vi "CPF_fast.vi"(1 "y":dbl=1.0, 2 "x":dbl=1.0) -> (0 "CPF Value":cdb=0.3047442052569335+0.2082189382028505i format="%#_12g")   [LabVIEW 2015]
panel:
  # "CPF algorithm"
  # "Fast CPF algorithm:\n  Computes the complex probability function using Humlicek's algorithm in\n  its first subregion (Source: 10.1016/0022-4073(82)90078-4) and using a\n  rational series with 24 terms in other subregions. (Source: \n  jstor.org/stable/2158232)\n\nStandard Input Parameters:\n-------------------- \nx  : Real part of input complex parameter\ny  : Imaginary part of input complex parameter\n\nThe function has one output:\n--------------------\n(1): Complex probability function"
  # "Output Section"
  # "Input Section"
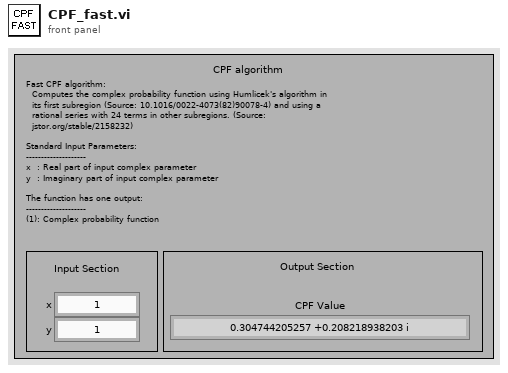
[diagram p1: front panel]
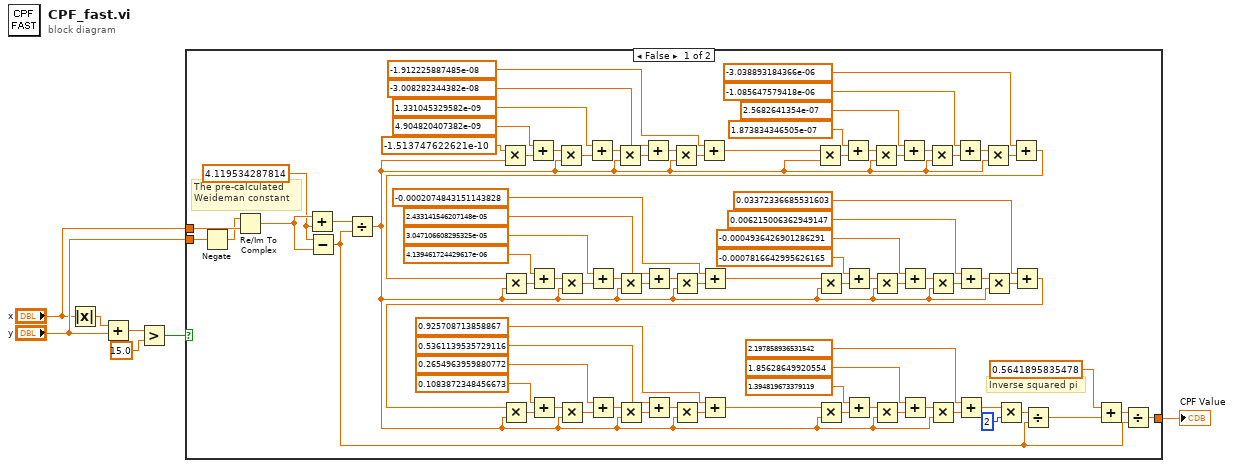
[diagram p0: block diagram]
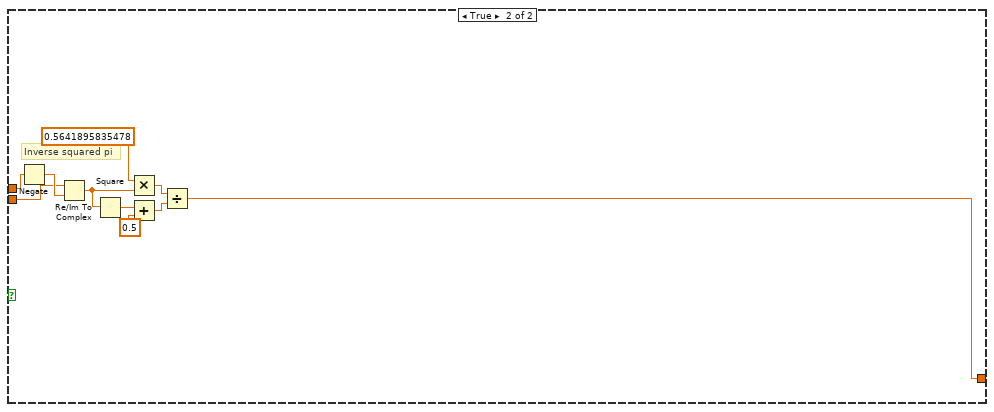
[diagram p2: hidden frame]
diagram:
  n1 = Absolute Value(x="x") -> (abs(x)=w4:dbl)
  n2 = Add(x=w4, y="y") -> (x+y=w3:dbl)
  n3 = Greater?(x=w3, y=15.0) -> (0:w5:bool)
  n4 = case shown="False" w5 {
    tunnel: "x" -> [w90 w101]
    tunnel: "y" -> [w91 w99]
    tunnel: [w77 w93] -> w1
    frame False {
      w87 = 4.119534287814 ("L")
      # "Inverse squared pi"
      # "The pre-calculated \nWeideman constant"
      n5 = Negate(x=w91) -> (-x=w89:dbl)
      n6 = Re/Im To Complex(1:w90, 2:w89) -> (0:w88:cdb)
      n7 = Add(x=w88, y=w87) -> (x+y=w86:cdb)
      n8 = Subtract(x=w87, y=w88) -> (x-y=w78:cdb)
      n9 = Divide(x=w86, y=w78) -> (x/y=w85:cdb)
      n10 = Multiply(x=-1.513747622621e-10, y=w85) -> (x*y=w76:cdb)
      n11 = Add(x=4.904820407382e-09, y=w76) -> (x+y=w75:cdb)
      n12 = Multiply(x=w75, y=w85) -> (x*y=w73:cdb)
      n13 = Add(x=1.331045329582e-09, y=w73) -> (x+y=w74:cdb)
      n14 = Multiply(x=w74, y=w85) -> (x*y=w70:cdb)
      n15 = Add(x=-3.008282344382e-08, y=w70) -> (x+y=w72:cdb)
      n16 = Multiply(x=w72, y=w85) -> (x*y=w71:cdb)
      n17 = Add(x=-1.912225887485e-08, y=w71) -> (x+y=w62:cdb)
      n18 = Multiply(x=w62, y=w85) -> (x*y=w69:cdb)
      n19 = Add(x=1.873834346505e-07, y=w69) -> (x+y=w68:cdb)
      n20 = Multiply(x=w68, y=w85) -> (x*y=w66:cdb)
      n21 = Add(x=2.5682641354e-07, y=w66) -> (x+y=w67:cdb)
      n22 = Multiply(x=w67, y=w85) -> (x*y=w63:cdb)
      n23 = Add(x=-1.085647579418e-06, y=w63) -> (x+y=w65:cdb)
      n24 = Multiply(x=w65, y=w85) -> (x*y=w64:cdb)
      n25 = Add(x=-3.038893184366e-06, y=w64) -> (x+y=w29:cdb)
      n26 = Multiply(x=w29, y=w85) -> (x*y=w52:cdb)
      n27 = Add(x=4.139461724429617e-06, y=w52) -> (x+y=w51:cdb)
      n28 = Multiply(x=w51, y=w85) -> (x*y=w49:cdb)
      n29 = Add(x=3.047106608295325e-05, y=w49) -> (x+y=w50:cdb)
      n30 = Multiply(x=w50, y=w85) -> (x*y=w46:cdb)
      n31 = Add(x=2.433141546207148e-05, y=w46) -> (x+y=w48:cdb)
      n32 = Multiply(x=w48, y=w85) -> (x*y=w47:cdb)
      n33 = Add(x=-0.0002074843151143828, y=w47) -> (x+y=w38:cdb)
      n34 = Multiply(x=w38, y=w85) -> (x*y=w45:cdb)
      n35 = Add(x=-0.0007816642995626165, y=w45) -> (x+y=w44:cdb)
      n36 = Multiply(x=w44, y=w85) -> (x*y=w42:cdb)
      n37 = Add(x=-0.0004936426901286291, y=w42) -> (x+y=w43:cdb)
      n38 = Multiply(x=w43, y=w85) -> (x*y=w39:cdb)
      n39 = Add(x=0.006215006362949147, y=w39) -> (x+y=w41:cdb)
      n40 = Multiply(x=w41, y=w85) -> (x*y=w40:cdb)
      n41 = Add(x=0.03372336685531603, y=w40) -> (x+y=w8:cdb)
      n42 = Multiply(x=w8, y=w85) -> (x*y=w28:cdb)
      n43 = Add(x=0.1083872348456673, y=w28) -> (x+y=w27:cdb)
      n44 = Multiply(x=w27, y=w85) -> (x*y=w25:cdb)
      n45 = Add(x=0.2654963959880772, y=w25) -> (x+y=w26:cdb)
      n46 = Multiply(x=w26, y=w85) -> (x*y=w22:cdb)
      n47 = Add(x=0.5361139535729116, y=w22) -> (x+y=w24:cdb)
      n48 = Multiply(x=w24, y=w85) -> (x*y=w23:cdb)
      n49 = Add(x=0.925708713858867, y=w23) -> (x+y=w16:cdb)
      n50 = Multiply(x=w16, y=w85) -> (x*y=w21:cdb)
      n51 = Add(x=1.394819673379119, y=w21) -> (x+y=w20:cdb)
      n52 = Multiply(x=w20, y=w85) -> (x*y=w18:cdb)
      n53 = Add(x=1.85628649920554, y=w18) -> (x+y=w19:cdb)
      n54 = Multiply(x=w19, y=w85) -> (x*y=w17:cdb)
      n55 = Add(x=2.197858936531542, y=w17) -> (x+y=w84:cdb)
      n56 = Multiply(x=w84, y=2) -> (x*y=w82:cdb)
      n57 = Divide(x=w82, y=w78) -> (x/y=w81:cdb)
      n58 = Add(x=0.5641895835478, y=w81) -> (x+y=w79:cdb)
      n59 = Divide(x=w79, y=w78) -> (x/y=w77:cdb)
    }
    frame True {
      # "Inverse squared pi"
      n60 = Negate(x=w101) -> (-x=w100:dbl)
      n61 = Re/Im To Complex(1:w100, 2:w99) -> (0:w98:cdb)
      n62 = Square(x=w98) -> (x^2=w97:cdb)
      n63 = Multiply(x=0.5641895835478, y=w98) -> (x*y=w94:cdb)
      n64 = Add(x=w97, y=0.5) -> (x+y=w95:cdb)
      n65 = Divide(x=w94, y=w95) -> (x/y=w93:cdb)
    }
  }
  "CPF Value" <- w1
